vi "Get Menu Tag & Item Name.vi"(8 "error in (no error)":errorcluster, 9 "Item Depth":i32, 10 "@ Locations":cluster{"Array":i32[]}, 11 "Menu Item Description":string) -> (0 "error out":errorcluster, 2 "Item Name":string, 3 "Menu Tag":string)   [LabVIEW 2019]
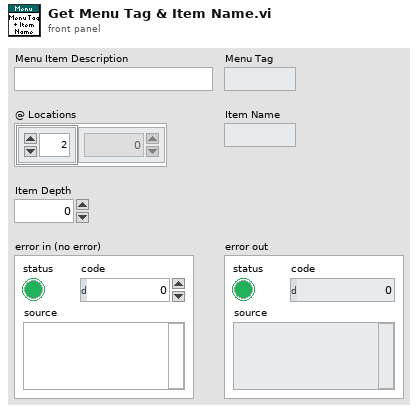
[diagram p1: front panel]
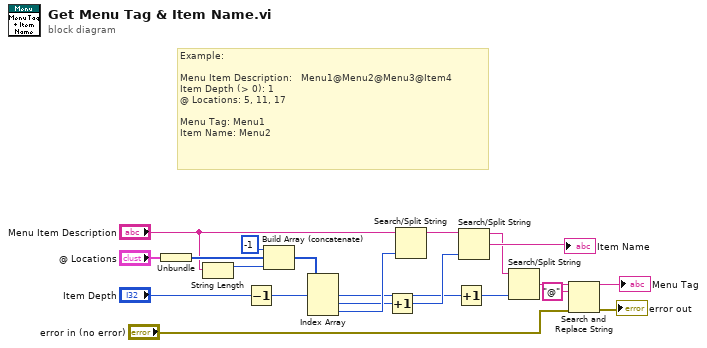
[diagram p0: block diagram]
diagram:
  # "Example:\n\nMenu Item Description:   Menu1@Menu2@Menu3@Item4\nItem Depth (> 0): 1\n@ Locations: 5, 11, 17\n\nMenu Tag: Menu1\nItem Name: Menu2"
  n1 = Unbundle("@ Locations") -> ("Array"=w20:i32[])
  n2 = String Length(string="Menu Item Description") -> (length=w17:i32)
  n3 = Decrement(x="Item Depth") -> (x-1=w16:i32)
  n4 = Build Array (concatenate)(-1 ("Item Depth"), w20, w17) -> (w19:i32[])
  n5 = Index Array(array=w19, index #1=w16) -> (element #1=w7:i32, element #2=w12:i32, element #3=w13:i32)  [unwired: 2 in]
  n6 = Increment(x=w12) -> (x+1=w10:i32)
  n7 = Search/Split String(string="Menu Item Description", offset (0)=w13) -> (substring before match=w11:string)  [unwired: 1 in, 2 out]
  n8 = Increment(x=w7) -> (x+1=w6:i32)
  n9 = Search/Split String(string=w11, offset (0)=w10) -> (substring before match=w8:string, match + rest of string=→"Item Name":string)  [unwired: 1 in, 1 out]
  n10 = Search/Split String(string=w8, offset (0)=w6) -> (match + rest of string=w5:string)  [unwired: 1 in, 2 out]
  n11 = Search and Replace String(input string=w5, search string="@", error in="error in (no error)") -> (result string=→"Menu Tag":string, error out=→"error out":errorcluster)  [unwired: 5 in, 2 out]
